vi "Decode Camera.vi"(8 "error in (no error)":errorcluster, 10 "unsigned byte array":u8[](array[numeric]), 11 "Vision Decoder in":refnum<class "Vision Decoder.lvclass">) -> (0 "error out":errorcluster, 3 "Vision Decoder out":refnum<class "Vision Decoder.lvclass">)   [LabVIEW 2022 SP3, in "Vision Decoder.lvlib" / "Vision Decoder.lvclass"]
uses:
  Vision Decoder.lvclass
  <vilib>/Analysis/Matrix/Datatypes/RealMatrix.ctl
  <vilib>/Analysis/Matrix/NI_Matrix.lvlib
  Controls/SSL Detection Robot.ctl
  Controls/SSL Detection Ball.ctl
  Controls/SSL Detection Frame.ctl
  Controls/SSL Geometry Camera Calibration.ctl
panel:
  out "Geometry Camera Calibration":T1
  out "Field Size":T2
  out "Detection Frame":T3 {"robots_blue"."height" format="%+4.3f"; "robots_blue"."pixel_y" format="%+4.3f"; "robots_blue"."pixel_x" format="%+4.3f"; "robots_blue"."orientation" format="%+4.3f"; "robots_blue"."y" format="%+4.3f"; "robots_blue"."confidence" format="%4.3f"; "robots_blue"."x" format="%+4.3f"; "robots_yellow"."height" format="%+4.3f"; "robots_yellow"."pixel_y" format="%+4.3f"; "robots_yellow"."pixel_x" format="%+4.3f"; "robots_yellow"."orientation" format="%+4.3f"; "robots_yellow"."y" format="%+4.3f"; "robots_yellow"."confidence" format="%4.3f"; "robots_yellow"."x" format="%+4.3f"}
  out "Empty Field Size?":bool
  out "Empty Information?":bool
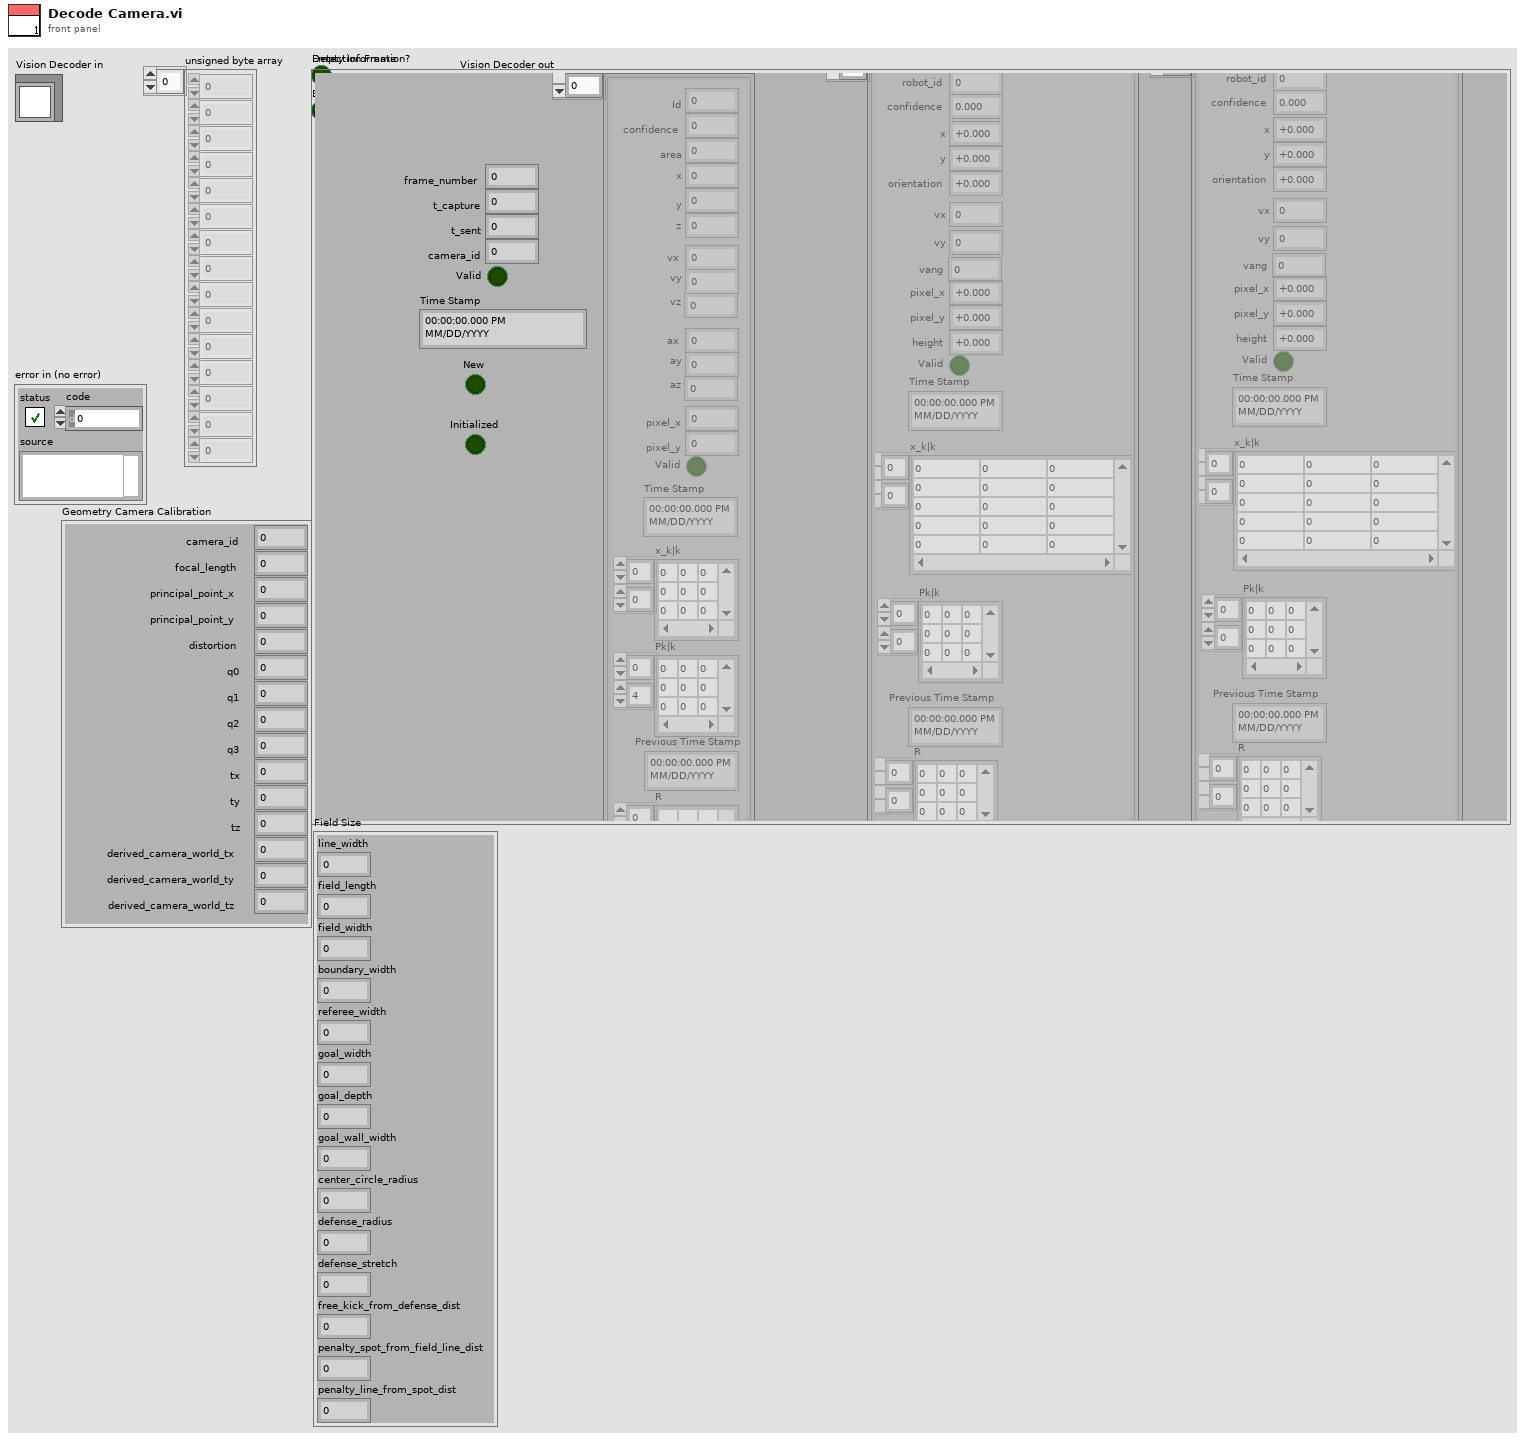
[diagram p1: front panel]
types:
  T1 = typedef "SSL Geometry Camera Calibration.ctl" = cluster{"camera_id":u32, "focal_length":sgl, "principal_point_x":sgl, "principal_point_y":sgl, "distortion":sgl, "q0":sgl, "q1":sgl, "q2":sgl, "q3":sgl, "tx":sgl, "ty":sgl, "tz":sgl, "derived_camera_world_tx":sgl, "derived_camera_world_ty":sgl, "derived_camera_world_tz":sgl}
  T2 = cluster{"line_width":u32, "field_length":u32, "field_width":u32, "boundary_width":u32, "referee_width":u32, "goal_width":u32, "goal_depth":u32, "goal_wall_width":u32, "center_circle_radius":u32, "defense_radius":u32, "defense_stretch":u32, "free_kick_from_defense_dist":u32, "penalty_spot_from_field_line_dist":u32, "penalty_line_from_spot_dist":u32}
  T3 = typedef "SSL Detection Frame.ctl" = cluster{"frame_number":u32, "t_capture":dbl, "t_sent":dbl, "camera_id":u32, "robots_yellow":T4[], "robots_blue":T4[], "balls":T6[], "Valid":bool, "Time Stamp":timestamp, "New":bool, "Initialized":bool}
  T4 = typedef "SSL Detection Robot.ctl" = cluster{"x":sgl, "robot_id":u32, "confidence":sgl, "y":sgl, "orientation":sgl, "pixel_x":sgl, "pixel_y":sgl, "height":sgl, "Valid":bool, "Time Stamp":timestamp, "x_k|k":T5, "Pk|k":T5, "Previous Time Stamp":timestamp, "R":T5, "vx":dbl, "vy":dbl, "vang":dbl}
  T5 = typedef "NI_Matrix.lvlib/RealMatrix.ctl" = dbl[][]
  T6 = typedef "SSL Detection Ball.ctl" = cluster{"x":sgl, "area":u32, "confidence":sgl, "y":sgl, "z":sgl, "pixel_x":sgl, "pixel_y":sgl, "Valid":bool, "Time Stamp":timestamp, "x_k|k":T5, "Pk|k":T5, "Id":u32, "Previous Time Stamp":timestamp, "R":T5, " vx":sgl, "vy":dbl, "vz":dbl, " ax":sgl, "ay":dbl, "az":dbl}
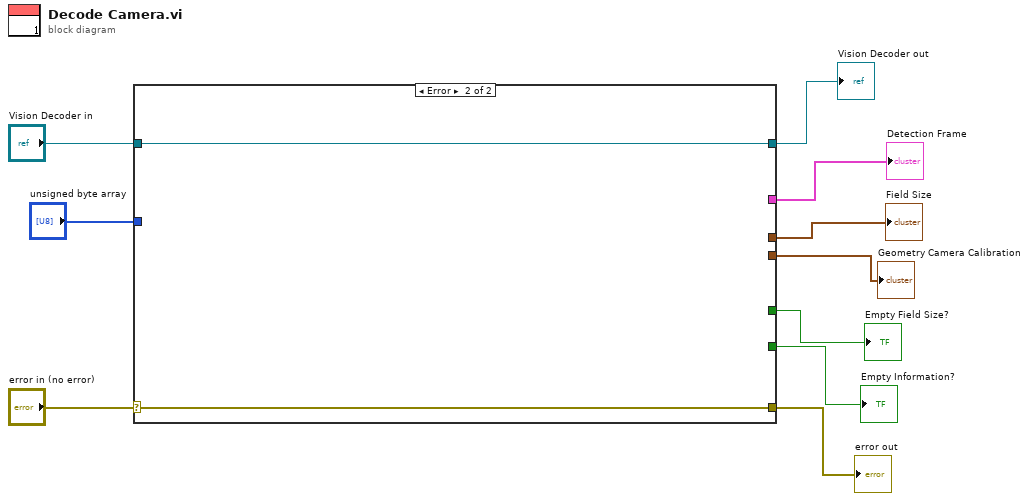
[diagram p0: block diagram]
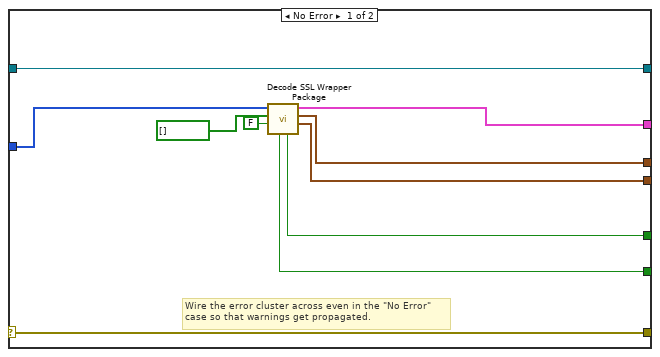
[diagram p2: hidden frame]
diagram:
  n1 = case shown="Error" "error in (no error)" {
    selector: "error in (no error)" -> [w19 w22]
    tunnel: [w19 w22] -> w9
    tunnel: [w20 w21] -> w7
    tunnel: "Vision Decoder in" -> [w20 w21]
    tunnel: "unsigned byte array" -> [w18 _]
    tunnel: [w17 _] -> w5
    tunnel: [w16 _] -> w4
    tunnel: [w15 _] -> w3
    tunnel: [w14 _] -> w2
    tunnel: [w13 _] -> w1
    frame No Error {
      # "Wire the error cluster across even in the \"No Error\"\ncase so that warnings get propagated."
      n2 = call "Decode SSL Wrapper Package.vi"("FIRASim?"=FALSE, "Ignore left/rigth?"=bool[] [], "unsigned byte array"=w18) -> ("Geometry Camera Calibration"=w13:T1, "Field Size"=w14:T2, "Detection Frame"=w15:T3, "Empty Field Size?"=w16:bool, "Empty Information?"=w17:bool)  [unwired: 3 in, 1 out]
    }
    frame Error {
    }
  }
  "error out" <- w9
  "Vision Decoder out" <- w7
  "Empty Information?" <- w5
  "Empty Field Size?" <- w4
  "Detection Frame" <- w3
  "Field Size" <- w2
  "Geometry Camera Calibration" <- w1
